vi "ApplyOverlayToVIs.vi"(6 "Total Iteration Progress":dbl, 7 "Project":refnum<vi>, 8 "error in (no error)":errorcluster, 9 "Hide Overlay?":bool, 10 "Overlay Icon":refnum<class "Icon.lvclass">, 11 "VIs":refnum<vi>[](array[refnum])) -> (0 "error out":errorcluster)   [LabVIEW 2016, in "NI_NPW_Icon Overlay.lvlib"]
uses:
  <resource>/dialog/NewProjectWizard/Icon Overlay/NI_NPW_Icon Overlay.lvlib
  <vilib>/LabVIEW Icon API/lv_icon/Classes/Icon/Icon.lvclass
  <vilib>/LabVIEW Icon API/API_User Layer Data.ctl
  <vilib>/Utility/miscctls.llb/LVPoint32TypeDef.ctl
  <vilib>/picture/picture.llb/imagedata.ctl
  <vilib>/LabVIEW Icon API/LabVIEW Icon API.lvlib
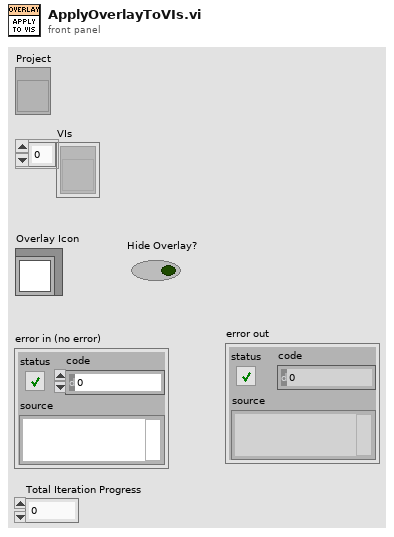
[diagram p1: front panel]
types:
  T1 = typedef "LabVIEW Icon API.lvlib/API_User Layer Data.ctl" = cluster{"Layer name":string, "Origin":T2, "Icon image data":T3}
  T2 = typedef "LVPoint32TypeDef.ctl" = cluster{"Horizontal":i32, "Vertical":i32}
  T3 = typedef "imagedata.ctl" = cluster{"image type":i32, "image depth":i32, "image":u8[], "mask":u8[], "colors":u32[], "Rectangle":cluster{"left":i16, "top":i16, "right":i16, "bottom":i16}}
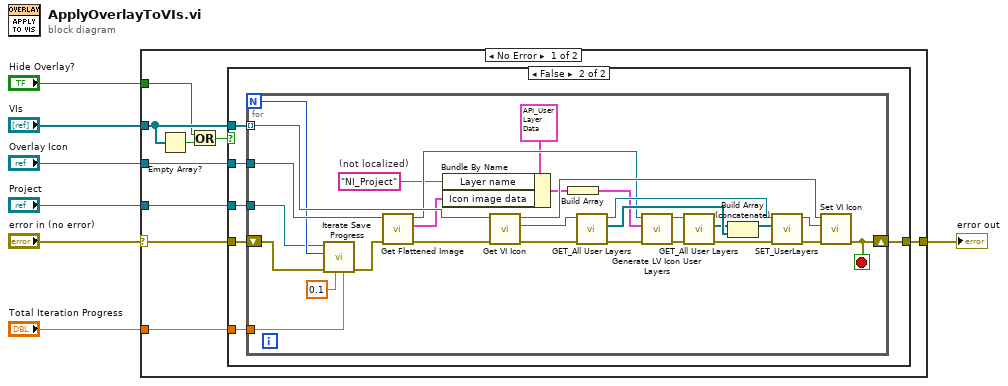
[diagram p0: block diagram]
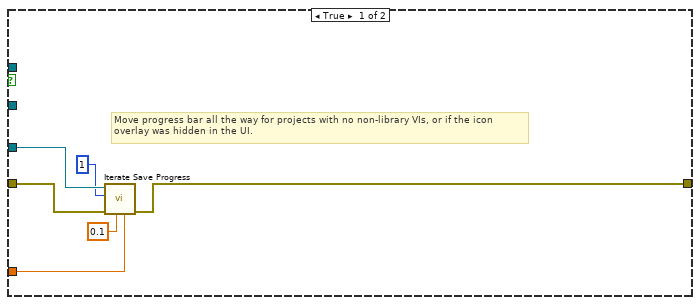
[diagram p2: hidden frame]
diagram:
  n1 = case shown="No Error" "error in (no error)" {
    selector: "error in (no error)" -> [w14 w58]
    tunnel: "VIs" -> [w11 _]
    tunnel: "Overlay Icon" -> [w16 _]
    tunnel: [w15 w58] -> w5
    tunnel: "Total Iteration Progress" -> [w13 _]
    tunnel: "Project" -> [w12 _]
    tunnel: "Hide Overlay?" -> [w8 _]
    frame No Error {
      n2 = Empty Array?(array=w11) -> (empty?=w10:bool)
      n3 = Or(x=w8, y=w10) -> (x .or. y?=w9:bool)
      n4 = case shown="False" w9 {
        tunnel: w16 -> [_ w28]
        tunnel: [w19 w27] -> w15
        tunnel: w14 -> [w22 w26]
        tunnel: w13 -> [w21 w25]
        tunnel: w12 -> [w20 w24]
        tunnel: w11 -> [_ w23]
        frame True {
          # "Move progress bar all the way for projects with no non-library VIs, or if the icon overlay was hidden in the UI."
          n5 = call <resource>:"Iterate Save Progress.vi"("Total Iteration Progress"=w21, "This Task's Percentage"=0.1, "error in (no error)"=w22, "Total Iterations (this task)"=1, "Project"=w20) -> ("error out"=w19:errorcluster)  [unwired: 6 in]
        }
        frame False {
          n6 = for {
            N -> [w35]
            tunnel: w23 -> [w57] mode=indexing
            tunnel: w28 -> [w50]
            shift-right: [w29] -> w27
            shift-left: w26 -> [w34]
            tunnel: w25 -> [w33]
            tunnel: w24 -> [w30]
            stop <- w29 stop-if-true
            w40 = "NI_Project"  # (not localized)
            n7 = call <resource>:"Iterate Save Progress.vi"("Total Iteration Progress"=w33, "This Task's Percentage"=0.1, "error in (no error)"=w34, "Total Iterations (this task)"=w35, "Project"=w30) -> ("error out"=w31:errorcluster)  [unwired: 6 in]
            n8 = call <vilib>:"Get Flattened Image.vi"("error in (no error)"=w31, "lv_icon.lvlib:Icon.lvclass in"=w50) -> ("error out"=w39:errorcluster, "Color Image"=w41:T3, "lv_icon.lvlib:Icon.lvclass out"=w45:refnum<class "Icon.lvclass">)  [unwired: 6 in, 1 out]
            n9 = Bundle By Name(cluster=T1 {"Layer name"="", "Origin"={"Horizontal"=0, "Vertical"=0}, "Icon image data"={"image type"=0, "image depth"=0, "image"=[], "mask"=[], "colors"=[], "Rectangle"={"left"=0, "top"=0, "right"=0, "bottom"=0}}} ("User layer"), "Layer name"=w40, "Icon image data"=w41) -> (w43:T1)
            n10 = call <vilib>:"Get VI Icon.vi"("error in (no error)"=w39, "VI Refnum in"=w57) -> ("error out"=w53:errorcluster, "Icon"=w52:refnum<class "Icon.lvclass">, "VI Refnum out"=w56:refnum<vi>)  [unwired: 7 in]
            n11 = Build Array(w43) -> (w42:T1[])
            n12 = call-dynamic "GET_All User Layers.vi"("error in (no error)"=w53, "Icon.lvclass in"=w52) -> ("error out"=w38:errorcluster, "User Layer"=w51:refnum<class "Layer.lvclass">[], "Icon.lvclass out"=w49:refnum<class "Icon.lvclass">)  [unwired: 7 in]
            n13 = call <vilib>:"Generate LV Icon User Layers.vi"("error in (no error)"=w38, "User layers"=w42, "Icon in"=w45) -> ("error out"=w48:errorcluster, "Icon out"=w47:refnum<class "Icon.lvclass">)  [unwired: 7 in]
            n14 = call-dynamic "GET_All User Layers.vi"("error in (no error)"=w48, "Icon.lvclass in"=w47) -> ("error out"=w37:errorcluster, "User Layer"=w46:refnum<class "Layer.lvclass">[])  [unwired: 7 in, 1 out]
            n15 = Build Array (concatenate)(w46, w51) -> (w54:refnum<class "Layer.lvclass">[])
            n16 = call-dynamic "SET_UserLayers.vi"("error in (no error)"=w37, "Layers"=w54, "Icon.lvclass in"=w49) -> ("error out"=w36:errorcluster, "Icon.lvclass out"=w55:refnum<class "Icon.lvclass">)  [unwired: 7 in]
            n17 = call <vilib>:"Set VI Icon.vi"("error in (no error)"=w36, "Icon"=w55, "VI Refnum in"=w56) -> ("error out"=w29:errorcluster)  [unwired: 7 in, 1 out]
          }
        }
      }
    }
    frame Error {
    }
  }
  "error out" <- w5
